vi "bats.parser.common.vi"(11 "BATS.Parser.State.Data in":T1={"BATS.Parser.States"=enum."Send.Command", "Hdr Length (U16)"=0, "MessageLength (U8)"=0, "MessageType (U8)"=0, "Time (U32)"=0, "Total Counter (U16)"=0, "Message Counter (U8)"=0, "i"=0, "Number.of.Tickers"=0, "Memory.Command"={"Read.Request"=FALSE, "Write.Request"=FALSE, "Address"=0, "Memory.Slot"={"Symbol"=0, "Base.Address"=0, "Num.of.Slots"=0}, "Read.Valid"=FALSE}}) -> (1 "MessageType (U8)":u8, 2 "Message Counter (U8)":u8, 3 "BATS.Parser.State.Data out":T1={"BATS.Parser.States"=enum."Send.Command", "Hdr Length (U16)"=0, "MessageLength (U8)"=0, "MessageType (U8)"=0, "Time (U32)"=0, "Total Counter (U16)"=0, "Message Counter (U8)"=0, "i"=0, "Number.of.Tickers"=0, "Memory.Command"={"Read.Request"=FALSE, "Write.Request"=FALSE, "Address"=0, "Memory.Slot"={"Symbol"=0, "Base.Address"=0, "Num.of.Slots"=0}, "Read.Valid"=FALSE}})   [LabVIEW 2022 SP3]
uses:
  bats.parser.state.data.ctl
  bats.parser.state.command.ctl
  memory/memory.command.ctl
  memory/memory.ticker.slot.ctl
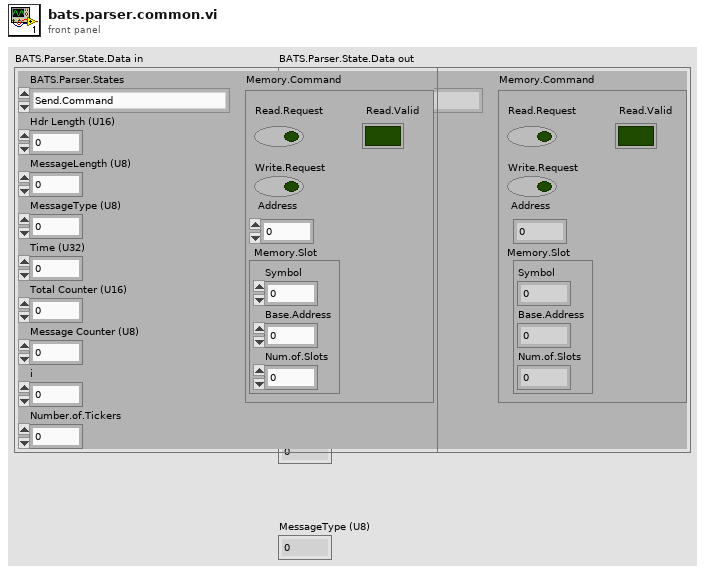
[diagram p1: front panel]
types:
  T1 = typedef "bats.parser.state.data.ctl" = cluster{"BATS.Parser.States":T2, "Hdr Length (U16)":u16, "MessageLength (U8)":u8, "MessageType (U8)":u8, "Time (U32)":u32, "Total Counter (U16)":u16, "Message Counter (U8)":u8, "i":u16, "Number.of.Tickers":u16, "Memory.Command":T3}
  T2 = typedef "bats.parser.state.command.ctl" = enum16{"No.Op", "Reset", "Configuration", "Filter", "Send.Command", "Read.Sequenced.Unit.Header", "Read.Msg.Type.and.Length", "Read.Time", "Read.Add.Order", "Read.Order.Executed", "Read.Reduce.Size", "Read.Modify.Order", "Read.Delete.Order"}
  T3 = typedef "memory.command.ctl" = cluster{"Read.Request":bool, "Write.Request":bool, "Address":u32, "Memory.Slot":T4, "Read.Valid":bool}
  T4 = typedef "Memory.Ticker.Slot.ctl" = cluster{"Symbol":u64, "Base.Address":u16, "Num.of.Slots":u16}
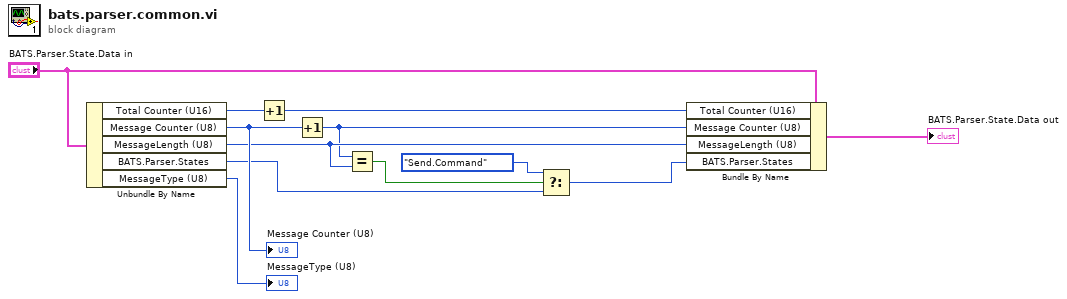
[diagram p0: block diagram]
diagram:
  n1 = Unbundle By Name("BATS.Parser.State.Data in") -> ("Total Counter (U16)"=w3:u16, "Message Counter (U8)"=w12:u8, "MessageLength (U8)"=w9:u8, "BATS.Parser.States"=w10:T2, "MessageType (U8)"=→"MessageType (U8)":u8)
  "Message Counter (U8)" <- w12
  n2 = Increment(x=w3) -> (x+1=w1:u16)
  n3 = Increment(x=w12) -> (x+1=w4:u8)
  n4 = Equal?(x=w4, y=w9) -> (x = y?=w5:bool)
  n5 = Select(t=bats.parser.state.command."Send.Command" ("BATS.Parser.States"), s=w5, f=w10) -> (s? t:f=w2:T2)
  n6 = Bundle By Name(cluster="BATS.Parser.State.Data in", "Total Counter (U16)"=w1, "Message Counter (U8)"=w4, "MessageLength (U8)"=w9, "BATS.Parser.States"=w2) -> (→"BATS.Parser.State.Data out":T1)
